vi "Qtegra_Control.vi"() -> ()   [LabVIEW 2015]
doc: "tesing the Qtegra Connection. This must be run on the local machine where Qtegra is installed.\nSeveral predefined commands can be send to qtegra."
panel:
  in  "command":string(combo)="GetMagnetDAC"
  out "answer":string
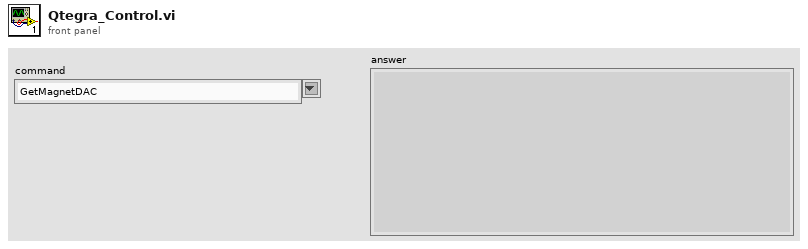
[diagram p1: front panel]
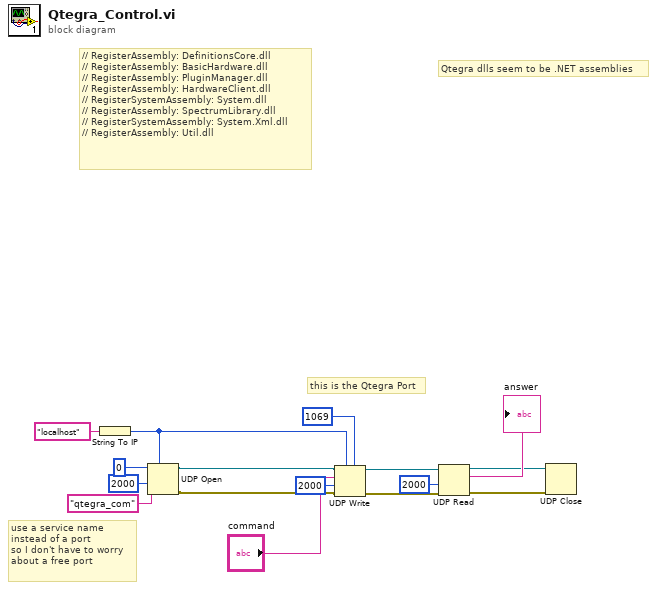
[diagram p0: block diagram]
diagram:
  # "use a service name\ninstead of a port\nso I don't have to worry\nabout a free port"
  # "this is the Qtegra Port"
  # "Qtegra dlls seem to be .NET assemblies"
  # "// RegisterAssembly: DefinitionsCore.dll\n// RegisterAssembly: BasicHardware.dll\n// RegisterAssembly: PluginManager.dll\n// RegisterAssembly: HardwareClient.dll\n// RegisterSystemAssembly: System.dll\n// RegisterAssembly: SpectrumLibrary.dll\n// RegisterSystemAssembly: System.Xml.dll\n// RegisterAssembly: Util.dll"
  n1 = String To IP(1:"localhost" ("name")) -> (0:w11:u32)
  n2 = UDP Open(7:w11, 9:2000 ("timeout ms (25000)"), 10:"qtegra_com" ("service name"), 11:u16 0 ("port")) -> (port=w13:refnum<k16>, 0:w12:errorcluster)  [unwired: 1 in, 1 out]
  n3 = UDP Write(address=w11, port or service name=u16 1069, connection ID=w13, data in="command", 8:w12, 9:2000 ("timeout ms (25000)")) -> (error out=w8:errorcluster, 3:w9:refnum<k16>)
  n4 = UDP Read(connection ID=w9, timeout ms (25000)=2000, 8:w8) -> (data out=→"answer":string, error out=w1:errorcluster, 3:w2:refnum<k16>)  [unwired: 1 in, 2 out]
  n5 = UDP Close(connection ID=w2, 8:w1) -> ()  [unwired: 2 out]
